vi "Andor_ProcessData.vi"(8 "error in (no error)":errorcluster caption="entrée d'erreur (pas d'erreur)", 10 "WaveBands":T1(array[cluster]) {"WB End" min=1 max=255 step=1; "WB Start" min=1 max=255 step=1}, 11 "Data":dbl[](array[numeric])) -> (0 "error out":errorcluster caption="sortie d'erreur", 3 "WB Cnts":dbl[](array[numeric]))   [LabVIEW 2019]
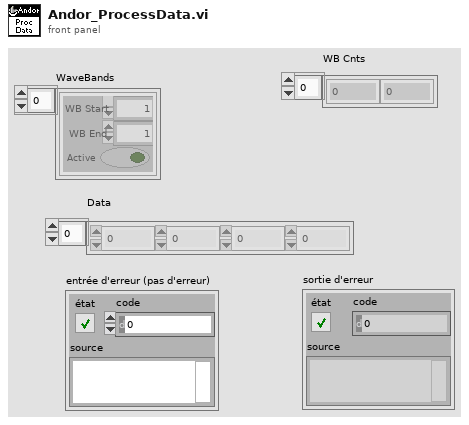
[diagram p1: front panel]
types:
  T1 = cluster{"WB Start":i32, "WB End":i32, "Active":bool}[]
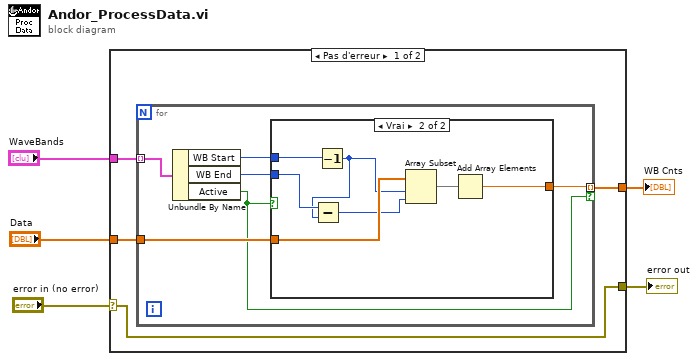
[diagram p0: block diagram]
diagram:
  n1 = case shown="Pas d'erreur" "error in (no error)" {
    selector: "error in (no error)" -> [w6 w23]
    tunnel: "WaveBands" -> [w9 _]
    tunnel: "Data" -> [w8 _]
    tunnel: [w7 _] -> w3
    tunnel: [w6 w23] -> w1
    frame No Error {
      n2 = for {
        tunnel: w9 -> [w15] mode=indexing
        tunnel: w8 -> [w14]
        tunnel: [w11] -> w7 mode=indexing if=w10
        n3 = Unbundle By Name(w15) -> ("WB Start"=w12:i32, "WB End"=w13:i32, "Active"=w10:bool)
        n4 = case shown="Vrai" w10 {
          tunnel: w14 -> [_ w22]
          tunnel: w13 -> [_ w21]
          tunnel: w12 -> [_ w20]
          tunnel: [_ w17] -> w11
          frame False {
          }
          frame True {
            n5 = Decrement(x=w20) -> (x-1=w16:i32)
            n6 = Subtract(x=w21, y=w16) -> (x-y=w19:i32)
            n7 = Array Subset(array=w22, index=w16, length=w19) -> (w18:dbl[])
            n8 = Add Array Elements(numeric array=w18) -> (sum=w17:dbl)
          }
        }
      }
    }
    frame Error {
    }
  }
  "WB Cnts" <- w3
  "error out" <- w1
